vi "onUnsubscribe.vi"(8 "error in (no error)":errorcluster, 10 "UNSUBSCRIBE":refnum<class "UNSUBSCRIBE.lvclass">, 11 "Client in":refnum<class "Client.lvclass">) -> (0 "error out":errorcluster, 3 "Client out":refnum<class "Client.lvclass">)   [LabVIEW 2013, in "MQTT Server.lvlib" / "Client.lvclass"]
uses:
  Client.lvclass
  Control Packets/UNSUBSCRIBE/UNSUBSCRIBE.lvclass
  MQTT_Base/MQTT_Base.lvclass
  Client.lvclass/Client.ctl
  Server/Session/Session.lvclass
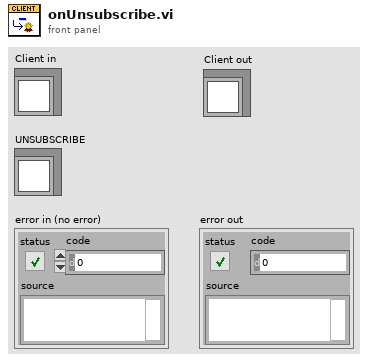
[diagram p1: front panel]
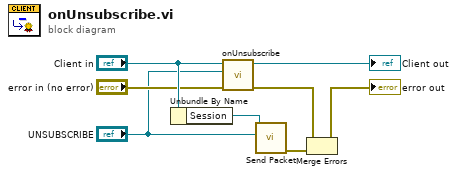
[diagram p0: block diagram]
diagram:
  n1 = Unbundle By Name("Client in") -> ("Session"=w8:refnum<class "Session.lvclass">)
  n2 = call-parent "onUnsubscribe.vi"("error in (no error)"="error in (no error)", "UNSUBSCRIBE"="UNSUBSCRIBE", "MQTT_Base in"="Client in") -> ("error out"=w6:errorcluster, "MQTT_Base out"=→"Client out":refnum<class "Client.lvclass">)  [unwired: 7 in]
  n3 = call "Send Packet.vi"("Packet"="UNSUBSCRIBE", "Session in"=w8) -> ("error out"=w7:errorcluster)  [unwired: 6 in, 3 out]
  n4 = Merge Errors(w6, w7) -> (→"error out":errorcluster)
